vi "Pos_Calculate box Global position.vi"(5 "Front Panel.PanelBounds":T1, 7 "Origin":T2, 8 "Error":errorcluster, 11 "Pane Position":T1) -> (0 "Error Out":errorcluster, 3 "Global Position Out":T1)   [LabVIEW 2015]
uses:
  <vilib>/Utility/miscctls.llb/LVRectTypeDef.ctl
  <vilib>/Utility/miscctls.llb/LVPointTypeDef.ctl
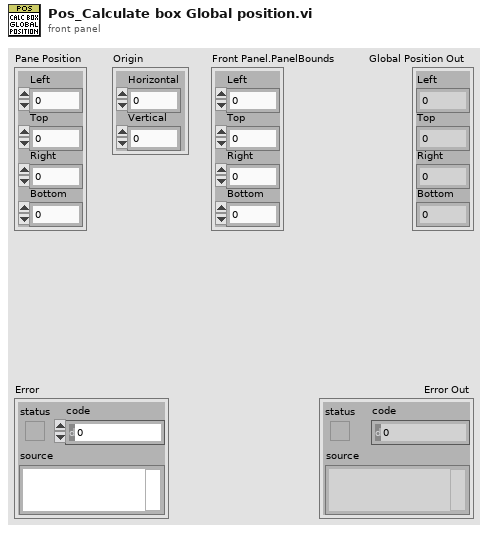
[diagram p1: front panel]
types:
  T1 = typedef "LVRectTypeDef.ctl" = cluster{"Left":i16, "Top":i16, "Right":i16, "Bottom":i16}
  T2 = typedef "LVPointTypeDef.ctl" = cluster{"Horizontal":i16, "Vertical":i16}
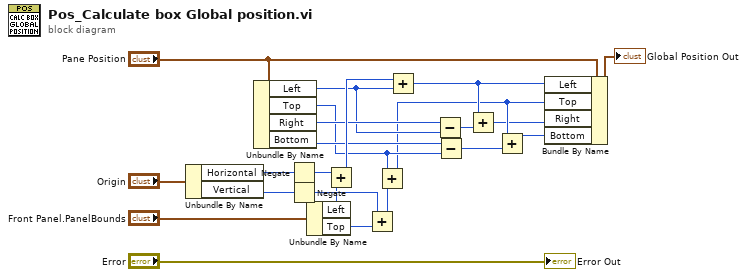
[diagram p0: block diagram]
diagram:
  n1 = Unbundle By Name("Origin") -> ("Horizontal"=w15:i16, "Vertical"=w16:i16)
  n2 = Unbundle By Name("Pane Position") -> ("Left"=w9:i16, "Top"=w7:i16, "Right"=w10:i16, "Bottom"=w8:i16)
  n3 = Negate(x=w15) -> (-x=w18:i16)
  n4 = Negate(x=w16) -> (-x=w19:i16)
  n5 = Unbundle By Name("Front Panel.PanelBounds") -> ("Left"=w17:i16, "Top"=w20:i16)
  n6 = Add(x=w18, y=w17) -> (x+y=w22:i16)
  n7 = Add(x=w19, y=w20) -> (x+y=w21:i16)
  n8 = Add(x=w7, y=w21) -> (x+y=w4:i16)
  n9 = Add(x=w22, y=w9) -> (x+y=w5:i16)
  n10 = Subtract(x=w10, y=w9) -> (x-y=w6:i16)
  n11 = Subtract(x=w8, y=w7) -> (x-y=w3:i16)
  n12 = Add(x=w5, y=w6) -> (x+y=w1:i16)
  n13 = Add(x=w4, y=w3) -> (x+y=w2:i16)
  n14 = Bundle By Name(cluster="Pane Position", "Left"=w5, "Top"=w4, "Right"=w1, "Bottom"=w2) -> (→"Global Position Out":T1)
  "Error Out" <- "Error"
